vi "FindSelfActorAttributes.vi"(11 "Actor":refnum<class "Actor.lvclass">) -> (3 "SelfActorAttributes":T1)   [LabVIEW 2020, in "jettl.lvlib"]
uses:
  jettl.lvlib
  Actor/Actor.lvclass
  Msg/Msg.lvclass
  MsgSet.ctl
  Msg.ctl
  PostSetup.ctl
  PreSetup.ctl
  Unified.ctl
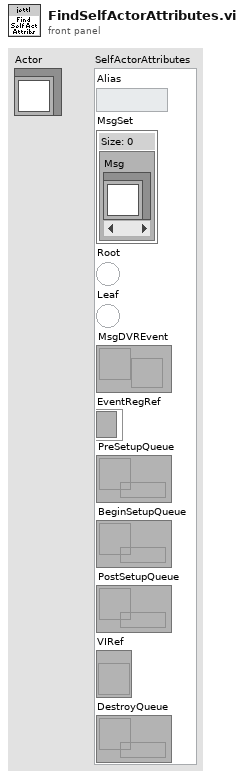
[diagram p1: front panel]
types:
  T1 = typedef "jettl.lvlib/Unified.ctl" = cluster{"Alias":string, "MsgSet":T2, "Root":bool, "Leaf":bool, "MsgDVREvent":refnum<user-event>, "EventRegRef":refnum<event-registration>, "PreSetupQueue":refnum<queue>, "BeginSetupQueue":refnum<queue>, "PostSetupQueue":refnum<queue>, "VIRef":refnum<vi>, "DestroyQueue":refnum<queue>}
  T2 = typedef "jettl.lvlib/MsgSet.ctl" = set{refnum<class "Msg.lvclass">}
  T3 = typedef "jettl.lvlib/Base.ctl" = cluster{"State":T4, "SelfUnified":T1, "ParentUnified":T1, "ChildUnifiedMap":T6}
  T4 = typedef "jettl.lvlib/State.ctl" = cluster{"Lifecycle":T5}
  T5 = typedef "jettl.lvlib/Lifecycle.ctl" = enum16{"Initializing", "SettingUp", "Starting", "Running", "Stopping", "TearingDown", "Terminated"}
  T6 = typedef "jettl.lvlib/ChildUnifiedMap.ctl" = map{string, T1}
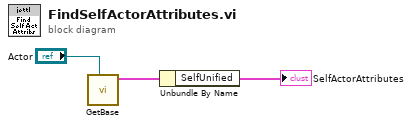
[diagram p0: block diagram]
diagram:
  n1 = call-dynamic "GetBase.vi"("Actor"="Actor") -> ("BaseActor"=w2:T3)  [unwired: 10 in]
  n2 = Unbundle By Name(w2) -> ("SelfUnified"=→"SelfActorAttributes":T1)
